vi "Append Multiple Waveforms.vi"(8 "error in (no error)":errorcluster, 10 "Waveform B []":waveform(dbl)[](array[waveform]), 11 "Waveforrm A []":waveform(dbl)[](array[waveform])) -> (0 "error out":errorcluster, 3 "Waveform out []":waveform(dbl)[](array[waveform]))   [LabVIEW 2019, in "Lockin.DAQ.lvclass"]
uses:
  Lockin.DAQ.lvclass
  <vilib>/Waveform/WDTOps.llb/WDT Append Waveforms DBL.vi
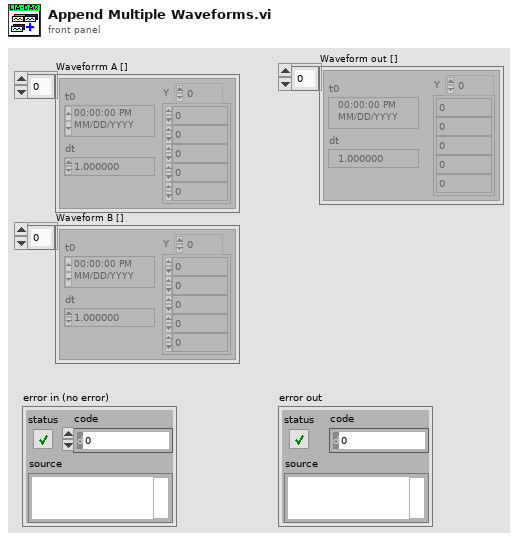
[diagram p1: front panel]
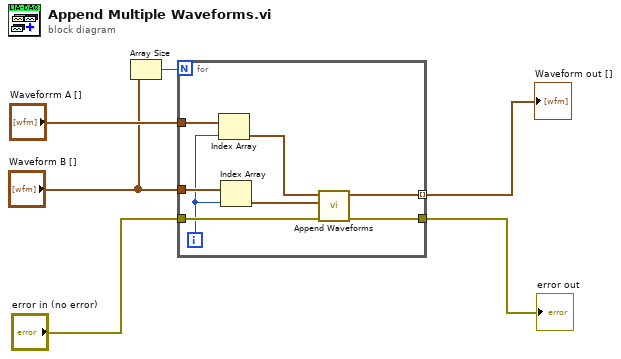
[diagram p0: block diagram]
diagram:
  n1 = Array Size(array="Waveform B []") -> (size(s)=w1:i32)
  n2 = for {
    N: w1 -> [_]
    tunnel: [w14] -> w5 mode=indexing
    tunnel: "error in (no error)" -> [w13]
    tunnel: [w12] -> w6
    tunnel: "Waveforrm A []" -> [w11]
    tunnel: "Waveform B []" -> [w9]
    i -> [w8]
    n3 = Index Array(array=w11, index=w8) -> (element=w10:waveform(dbl))
    n4 = Index Array(array=w9, index=w8) -> (element=w7:waveform(dbl))
    n5 = call-poly <vilib>:"Append Waveforms.vi"("error in (no error)"=w13, "waveform B"=w7, "waveform A"=w10) -> ("error out"=w12:errorcluster, "waveform out"=w14:waveform(dbl))  [unwired: 7 in]
  }
  "error out" <- w6
  "Waveform out []" <- w5
